vi "from string.vi"(8 "error in":errorcluster, 9 "data":string, 10 "version":string, 11 "bin datalogger configuration in":refnum<class "Binary datalogger configuration.lvclass">) -> (0 "error out":errorcluster, 3 "bin datalogger configuration out":refnum<class "Binary datalogger configuration.lvclass">)   [LabVIEW 2013, in "Binary datalogger configuration.lvclass"]
doc: "Provides an interface for loading a module configuration from a file or other serialized data source. It is recommended that all children of this class store data in two sets--data required for its own initialization, and any data required for parent initialization--and that each implementation uses the <b>Call Parent Method</b> primitive to de-serialize parent information. As a result, it is expected that every module configuration class calls <b>component configuration.lvclass:From String.vi</b>."
uses:
  Binary datalogger configuration.lvclass
  <vilib>/NI/Tag Bus Module Framework/channel/TBM channel.lvclass
  <vilib>/NI/Tag Bus Module Framework/module configuration/TBM module configuration.lvclass
  Binary datalogger configuration.lvclass/Binary datalogger configuration.ctl
  <vilib>/NI/Configuration Framework/serializable configuration/NISE_CEF_serializable configuration.lvclass
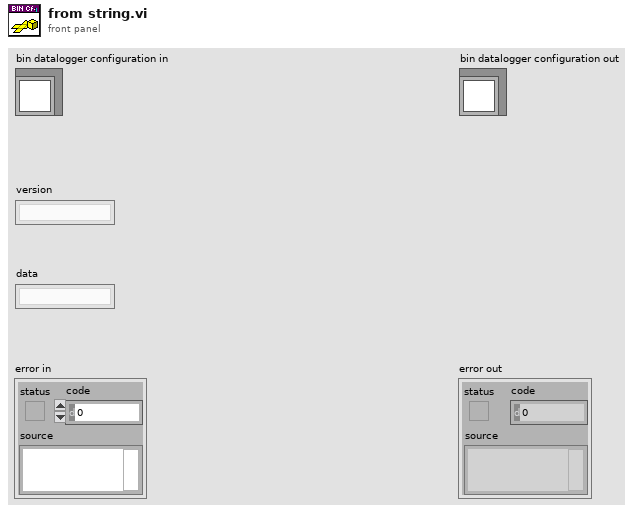
[diagram p1: front panel]
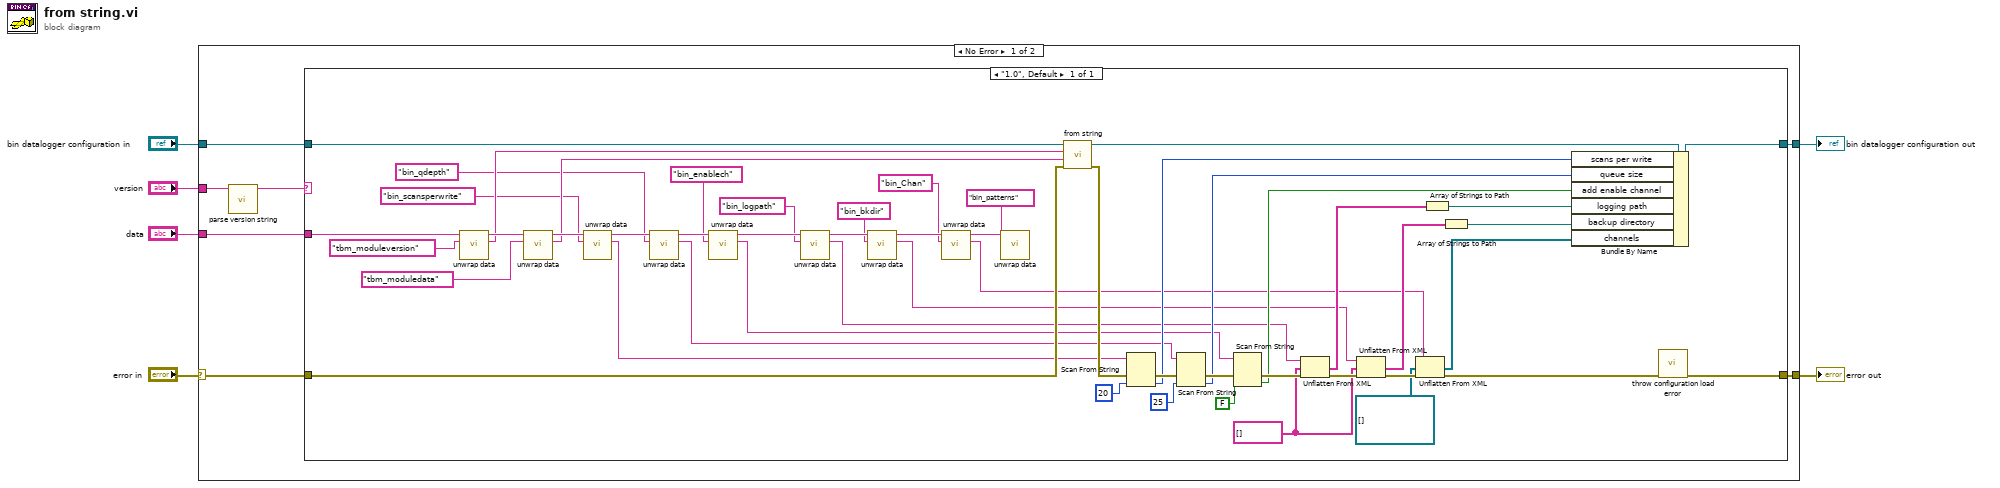
[diagram p0: block diagram]
diagram:
  n1 = case shown="No Error" "error in" {
    selector: "error in" -> [w7 w66]
    tunnel: "data" -> [w13 _]
    tunnel: "bin datalogger configuration in" -> [w12 w65]
    tunnel: [w11 w65] -> w5
    tunnel: [w10 w66] -> w4
    tunnel: "version" -> [w9 _]
    frame No Error {
      n2 = call <vilib>:"parse version string.vi"("full version"=w9) -> ("major.minor version"=w8:string)  [unwired: 7 in, 3 out]
      n3 = case shown="\"1.0\", Default" w8 {
        tunnel: w13 -> [w45]
        tunnel: w7 -> [w61]
        tunnel: w12 -> [w64]
        tunnel: [w63] -> w11
        tunnel: [w18] -> w10
        frame "1.0", Default {
          w14 = string[] [] ("array of strings")
          n4 = call <vilib>:"unwrap data.vi"("identifier"="tbm_moduleversion" ("additional identifier"), "data to unwrap"=w45) -> ("unwrapped data"=w44:string, "remaining string"=w51:string)  [unwired: 8 in]
          n5 = call <vilib>:"unwrap data.vi"("identifier"="tbm_moduledata" ("additional identifier"), "data to unwrap"=w51) -> ("unwrapped data"=w43:string, "remaining string"=w48:string)  [unwired: 8 in]
          n6 = call <vilib>:"unwrap data.vi"("identifier"="bin_scansperwrite" ("additional identifier"), "data to unwrap"=w48) -> ("unwrapped data"=w29:string, "remaining string"=w47:string)  [unwired: 8 in]
          n7 = call <vilib>:"unwrap data.vi"("identifier"="bin_qdepth" ("additional identifier"), "data to unwrap"=w47) -> ("unwrapped data"=w27:string, "remaining string"=w46:string)  [unwired: 8 in]
          n8 = call <vilib>:"unwrap data.vi"("identifier"="bin_enablech" ("additional identifier"), "data to unwrap"=w46) -> ("unwrapped data"=w25:string, "remaining string"=w33:string)  [unwired: 8 in]
          n9 = call <vilib>:"unwrap data.vi"("identifier"="bin_logpath" ("additional identifier"), "data to unwrap"=w33) -> ("unwrapped data"=w23:string, "remaining string"=w32:string)  [unwired: 8 in]
          n10 = call <vilib>:"unwrap data.vi"("identifier"="bin_bkdir" ("additional identifier"), "data to unwrap"=w32) -> ("unwrapped data"=w22:string, "remaining string"=w31:string)  [unwired: 8 in]
          n11 = call <vilib>:"unwrap data.vi"("identifier"="bin_Chan" ("additional identifier"), "data to unwrap"=w31) -> ("unwrapped data"=w21:string, "remaining string"=w17:string)  [unwired: 8 in]
          n12 = call <vilib>:"unwrap data.vi"("identifier"="bin_patterns", "data to unwrap"=w17) -> ()  [unwired: 8 in, 2 out]
          n13 = call-parent "from string.vi"("error in"=w61, "data"=w43, "version"=w44, "module configuration in"=w64) -> ("error out"=w62:errorcluster, "module configuration out"=w60:refnum<class "Binary datalogger configuration.lvclass">)  [unwired: 6 in]
          n14 = Scan From String(input string=w29, error in=w62, default 1=u16 20 ("scans per write")) -> (error out=w40:errorcluster, output 1=w34:u16)  [unwired: 2 in, 2 out]
          n15 = Scan From String(input string=w27, error in=w40, default 1=u16 25 ("queue size")) -> (error out=w41:errorcluster, output 1=w36:u16)  [unwired: 2 in, 2 out]
          n16 = Scan From String(input string=w25, error in=w41, default 1=FALSE ("add enable channel")) -> (error out=w42:errorcluster, output 1=w38:bool)  [unwired: 2 in, 2 out]
          n17 = Unflatten From XML(xml string=w23, type=w14, error in (no error)=w42) -> (value=w52:string[], error out=w56:errorcluster)
          n18 = Unflatten From XML(xml string=w22, type=w14, error in (no error)=w56) -> (value=w53:string[], error out=w57:errorcluster)
          n19 = Unflatten From XML(xml string=w21, type=refnum<class "TBM channel.lvclass">[] [] ("channels"), error in (no error)=w57) -> (value=w54:refnum<class "TBM channel.lvclass">[], error out=w15:errorcluster)
          n20 = Array of Strings to Path(0:w52) -> (2:w59:path)  [unwired: 1 in]
          n21 = Array of Strings to Path(0:w53) -> (2:w58:path)  [unwired: 1 in]
          n22 = Bundle By Name(cluster=w60, "scans per write"=w34, "queue size"=w36, "add enable channel"=w38, "logging path"=w59, "backup directory"=w58, "channels"=w54) -> (w63:refnum<class "Binary datalogger configuration.lvclass">)
          n23 = call <vilib>:"throw configuration load error.vi"("error in"=w15) -> ("error out"=w18:errorcluster)  [unwired: 10 in]
        }
      }
    }
    frame Error {
    }
  }
  "error out" <- w4
  "bin datalogger configuration out" <- w5
